vi "SubVI - Send Report Files.vi"(8 "error in (no error)":errorcluster, 11 "file path (use dialog)":path) -> (0 "error out":errorcluster)   [LabVIEW 2017]
panel:
  out "x-y":dbl
  out "Timer":u32
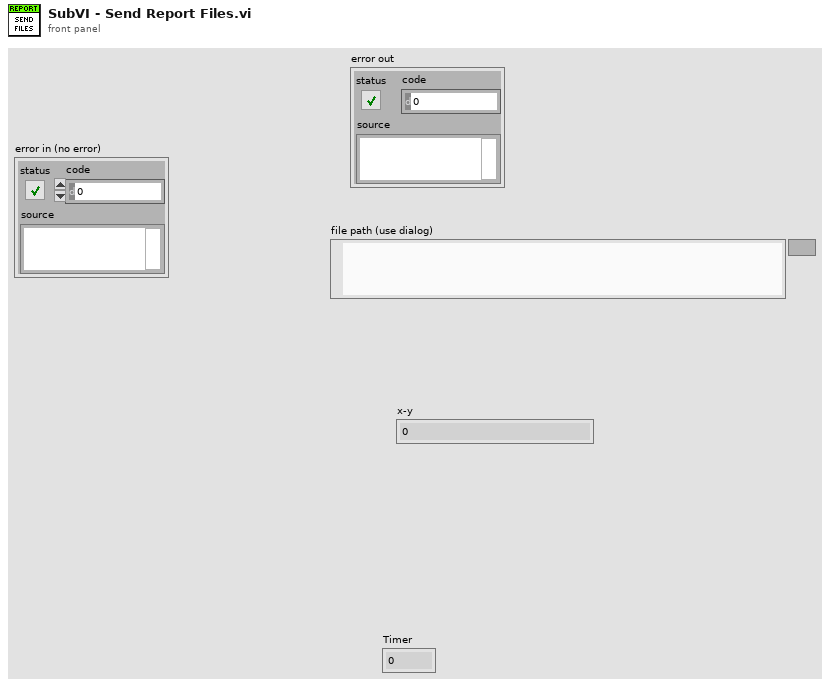
[diagram p1: front panel]
types:
  T1 = enum16{"open", "replace", "create", "open or create", "replace or create", "replace or create with confirmation"}
  T2 = enum16{"big-endian, network order", "native, host order", "little-endian"}
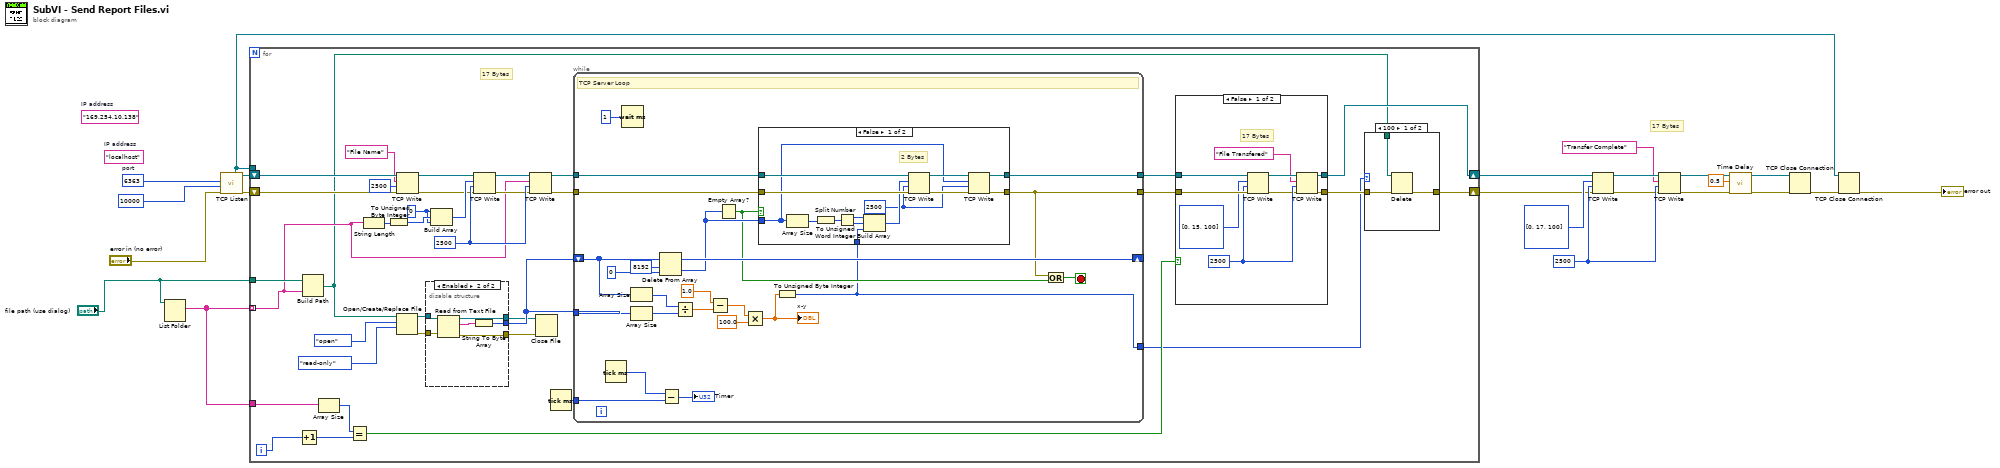
[diagram p0: block diagram]
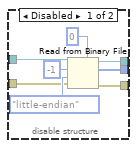
[diagram p3: hidden frame]
diagram:
  (unwired) "169.254.10.138"  # IP address
  w17 = 2500 ("timeout ms (25000)")
  w21 = u16 6363  # port
  (unwired) "localhost"  # IP address
  # "17 Bytes"
  n1 = List Folder(path="file path (use dialog)") -> (filenames=w4:string[])  [unwired: 3 in, 3 out]
  n2 = call <vilib>:"TCP Listen.vi"("error in (no error)"="error in (no error)", "timeout ms (wait forever: -1)"=10000, "port"=w21) -> ("error out"=w18:errorcluster, "connection ID"=w19:refnum<k5>, "listener ID"=w3:refnum<k5>)  [unwired: 4 in, 2 out]
  n3 = for {
    tunnel: "file path (use dialog)" -> [w32]
    shift-right: [w56] -> w10
    shift-left: w19 -> [w58]
    shift-right: [w25] -> w9
    shift-left: w18 -> [w57]
    tunnel: w4 -> [w31] mode=indexing
    tunnel: w4 -> [w30]
    tunnel: w3 -> [_]
    i -> [w28]
    w45 = 2500 ("timeout ms (25000)")
    w37 = u8 0
    # "17 Bytes"
    n4 = Increment(x=w28) -> (x+1=w26:i32)
    n5 = Build Path(base path=w32, name or relative path=w31) -> (appended path=w24:path)
    n6 = Array Size(array=w30) -> (size(s)=w29:i32)
    n7 = Equal?(x=w29, y=w26) -> (x = y?=w27:bool)
    n8 = String Length(string=w31) -> (length=w39:i32)
    n9 = To Unsigned Byte Integer(number=w39) -> (unsigned 8bit integer=w38:u8)
    n10 = Open/Create/Replace File(file path (use dialog)=w24, operation (0:open)=T1."open", access (0:read/write)=enum16{"read/write", "read-only", "write-only"}."read-only") -> (refnum out=w53:refnum<file>, error out=w52:errorcluster)  [unwired: 3 in, 1 out]
    n11 = TCP Write(connection ID=w58, data in="File Name", error in (no error)=w57, 9:2500 ("timeout ms (25000)")) -> (connection ID out=w36:refnum<k5>, error out=w35:errorcluster)  [unwired: 1 out]
    n12 = disable-structure shown="Enabled" {
      disable-tunnel: w53 -> [w67 w75]
      disable-tunnel: w52 -> [w66 w76]
      disable-tunnel: [w65 w71] -> w51
      disable-tunnel: [w64 w74] -> w50
      disable-tunnel: [w63 w73] -> w49
      frame Disabled {
        n13 = Read from Binary File(5:u8 0, 8:w66, 9:T2."little-endian" ("byte order (0:big-endian, network order)"), 10:-1 ("count (1)"), 11:w67) -> (0:w63:errorcluster, 2:w65:u8[], 3:w64:refnum<file>)  [unwired: 1 in, 1 out]
      }
      frame Enabled {
        n14 = Read from Text File(file (use dialog)=w75, error in=w76) -> (refnum out=w74:refnum<file>, text=w72:string, error out=w73:errorcluster)  [unwired: 2 in, 1 out]
        n15 = String To Byte Array(string=w72) -> (unsigned byte array=w71:u8[])
      }
    }
    n16 = Build Array(w37, w38, w37) -> (w40:u8[])
    n17 = TCP Write(connection ID=w36, data in=w40, error in (no error)=w35, 9:w45) -> (connection ID out=w43:refnum<k5>, error out=w44:errorcluster)  [unwired: 1 out]
    n18 = TCP Write(connection ID=w43, data in=w31, error in (no error)=w44, 9:w45) -> (connection ID out=w42:refnum<k5>, error out=w41:errorcluster)  [unwired: 1 out]
    n19 = Close File(refnum=w50, error in=w49) -> ()  [unwired: 2 out]
    n20 = Tick Count (ms)() -> (millisecond timer value=w48:u32)
    n21 = while {
      tunnel: w41 -> [w103]
      tunnel: w42 -> [w104]
      tunnel: [w110] -> w47
      tunnel: [w105] -> w46
      shift-right: [w107] -> _
      shift-left: w51 -> [w99]
      tunnel: w51 -> [w100]
      tunnel: w48 -> [w91]
      tunnel: [w88] -> w22
      stop <- w106 stop-if-true
      # "TCP Server Loop"
      n22 = Tick Count (ms)() -> (millisecond timer value=w92:u32)
      n23 = Wait (ms)(milliseconds to wait=u32 1) -> ()  [unwired: 1 out]
      n24 = Array Size(array=w99) -> (size(s)=w97:i32)
      n25 = Array Size(array=w100) -> (size(s)=w98:i32)
      n26 = Delete From Array(array=w99, length=8192, index=0) -> (deleted portion=w102:u8[], array with subset deleted=w107:u8[])
      n27 = Subtract(x=w92, y=w91) -> (x-y=→"Timer":u32)
      n28 = Divide(x=w97, y=w98) -> (x/y=w95:dbl)
      n29 = Subtract(x=1.0, y=w95) -> (x-y=w94:dbl)
      n30 = Empty Array?(array=w102) -> (empty?=w101:bool)
      n31 = Multiply(x=w94, y=100.0) -> (x*y=w89:dbl)
      "x-y" <- w89
      n32 = To Unsigned Byte Integer(number=w89) -> (unsigned 8bit integer=w88:u8)
      n33 = case shown="False" w101 {
        tunnel: [w125 w127] -> w110
        tunnel: [w124 w126] -> w105
        tunnel: w104 -> [w123 w127]
        tunnel: w103 -> [w121 w126]
        tunnel: w102 -> [w119 _]
        tunnel: w88 -> [w112 _]
        frame False {
          w113 = 2500 ("timeout ms (25000)")
          # "2 Bytes"
          n34 = Array Size(array=w119) -> (size(s)=w118:i32)
          n35 = To Unsigned Word Integer(number=w118) -> (unsigned 16bit integer=w117:u16)
          n36 = Split Number(x=w117) -> (hi(x)=w116:u8, lo(x)=w115:u8)
          n37 = Build Array(w116, w115, w112) -> (w114:u8[])
          n38 = TCP Write(connection ID=w123, data in=w114, error in (no error)=w121, 9:w113) -> (connection ID out=w122:refnum<k5>, error out=w120:errorcluster)  [unwired: 1 out]
          n39 = TCP Write(connection ID=w122, data in=w119, error in (no error)=w120, 9:w113) -> (connection ID out=w125:refnum<k5>, error out=w124:errorcluster)  [unwired: 1 out]
        }
        frame True {
        }
      }
      n40 = Or(x=w105, y=w101) -> (x .or. y?=w106:bool)
    }
    n41 = case shown="False" w27 {
      tunnel: [w85 w86] -> w56
      tunnel: [w84 w87] -> w23
      tunnel: w47 -> [w83 w86]
      tunnel: w46 -> [w82 w87]
      frame False {
        w81 = 2500 ("timeout ms (25000)")
        # "17 Bytes"
        n42 = TCP Write(connection ID=w83, data in=u8[] [0, 15, 100], error in (no error)=w82, 9:w81) -> (connection ID out=w79:refnum<k5>, error out=w80:errorcluster)  [unwired: 1 out]
        n43 = TCP Write(connection ID=w79, data in="File Transfered", error in (no error)=w80, 9:w81) -> (connection ID out=w85:refnum<k5>, error out=w84:errorcluster)  [unwired: 1 out]
      }
      frame True {
      }
    }
    n44 = case shown="100" w22 {
      tunnel: w23 -> [w61 w62]
      tunnel: [w60 w62] -> w25
      tunnel: w24 -> [w59 _]
      frame 100 {
        n45 = Delete(path (use dialog)=w59, error in=w61) -> (error out=w60:errorcluster)  [unwired: 3 in, 2 out]
      }
      frame 1, Default {
      }
    }
  }
  n46 = TCP Write(connection ID=w10, data in=u8[] [0, 17, 100], error in (no error)=w9, 9:w17) -> (connection ID out=w15:refnum<k5>, error out=w16:errorcluster)  [unwired: 1 out]
  n47 = TCP Write(connection ID=w15, data in="Transfer Complete", error in (no error)=w16, 9:w17) -> (connection ID out=w8:refnum<k5>, error out=w13:errorcluster)  [unwired: 1 out]
  n48 = call "Time Delay"("error in (no error)"=w13, "Delay Time (s)"=0.5) -> ("error out"=w7:errorcluster)  [unwired: 9 in]
  n49 = TCP Close Connection(connection ID=w8, error in (no error)=w7) -> (error out=w2:errorcluster)  [unwired: 1 in, 1 out]
  n50 = TCP Close Connection(connection ID=w3, error in (no error)=w2) -> (error out=→"error out":errorcluster)  [unwired: 1 in, 1 out]
